vi "OE2031&OE2041_Configure Auto_Setting.vi"(7 "OE2041_Auto Setting":T1, 8 "Error in (no error)":errorcluster caption="error out（no error）", 9 "Remote Mode":u16(ring) items=["USB"=0, "RS232"=1, "Ethernet"=3], 10 "Connection ID in":refnum<k5>, 11 "VISA resource name":refnum<visa-resource-name>) -> (0 "Error out":errorcluster caption="error out", 1 "Output String":string, 2 "Connection ID out":refnum<k5>, 3 "VISA resource  out":refnum<visa-resource-name>)   [LabVIEW 2011]
panel:
  out "字符串":string
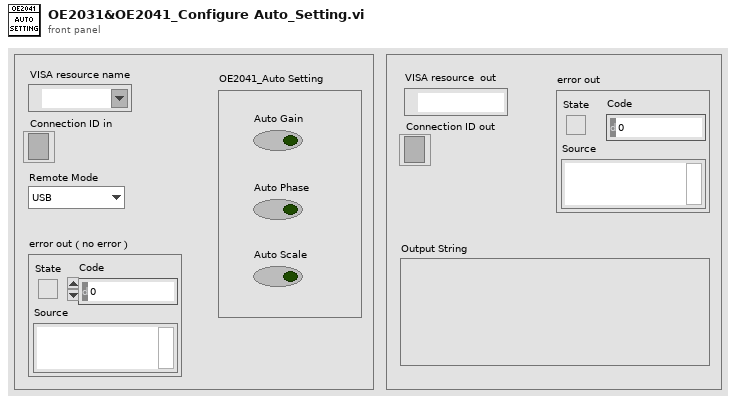
[diagram p1: front panel]
types:
  T1 = cluster{"Auto Gain":bool, "Auto Phase":bool, "Auto Scale":bool}
  T2 = enum16{"ISRC", "IGND", "ICPL", "ILIN", "PHAS", "FMOD", "RSLP", "FREQ", "SWPT", "SLLM", "SULM", "SSLL", "SSLG", "STLM", "SWRM", "IRNG", "SENS", "RMOD", "OFLT", "OFSL", "SYNC", "DMOD", "HARM", "DARB", "SWVT", "SLVL", "SVLL", "SVUL", "SVSL", "SVSG", "SVTM", "SVRM", "RALL", "SNAP", "OUTP", "OAUX", "COUT", "CAUX", "COFP", "CEXP", "FPOP", "OEXP", "*IDN", "*RST", "OVLD", "INOV", "GNOV", "*PLL", "SSET", "RSET", "AGAN", "APHS", "ARSV", "ASCL", "EQCD", "EQCS", "SPED", "SRAT", "SLEN", "SSLE", "STRG", "SPRM", "STRD", "PAUS", "REST", "SPTS", "TRCA", "TEMP", "RSTU", "IHNZ", "DEQU", "SADD", "ARNG", "CSPE", "ISRCD", "IGNDD", "ICPLD", "ILIND", "PHASD", "FMODD", "RSLPD", "FREQD", "SWPTD", "SLLMD", "SULMD", "SSLLD", "SSLGD", "STLMD", "SWRMD", "SENSD", "RMODD", "OFLTD", "OFSLD", "SYNCD", "HARMD", "EQCDD", "EQCSD", "SNAPD", "OUTPD", "SWVTD", "SLVLD", "SVLLD", "SVULD", "SVSLD", "SVSGD", "SVTMD", "SVRMD", "SVDCD", "ARSVD", "AGAND", "APHSD", "ASCLD", "FPOPD", "CAUXD", "OEXPD", "SPEDD", "SRATD", "SLEND", "SSLED", "STRGD", "SPRMD", "STRDD", "PAUSD", "RESTD", "SPTSD", "TRCAD", "*IDND", "*RSTD", "INOVD", "GNOVD", "*PLLD", "SSETD", "RSETD"}
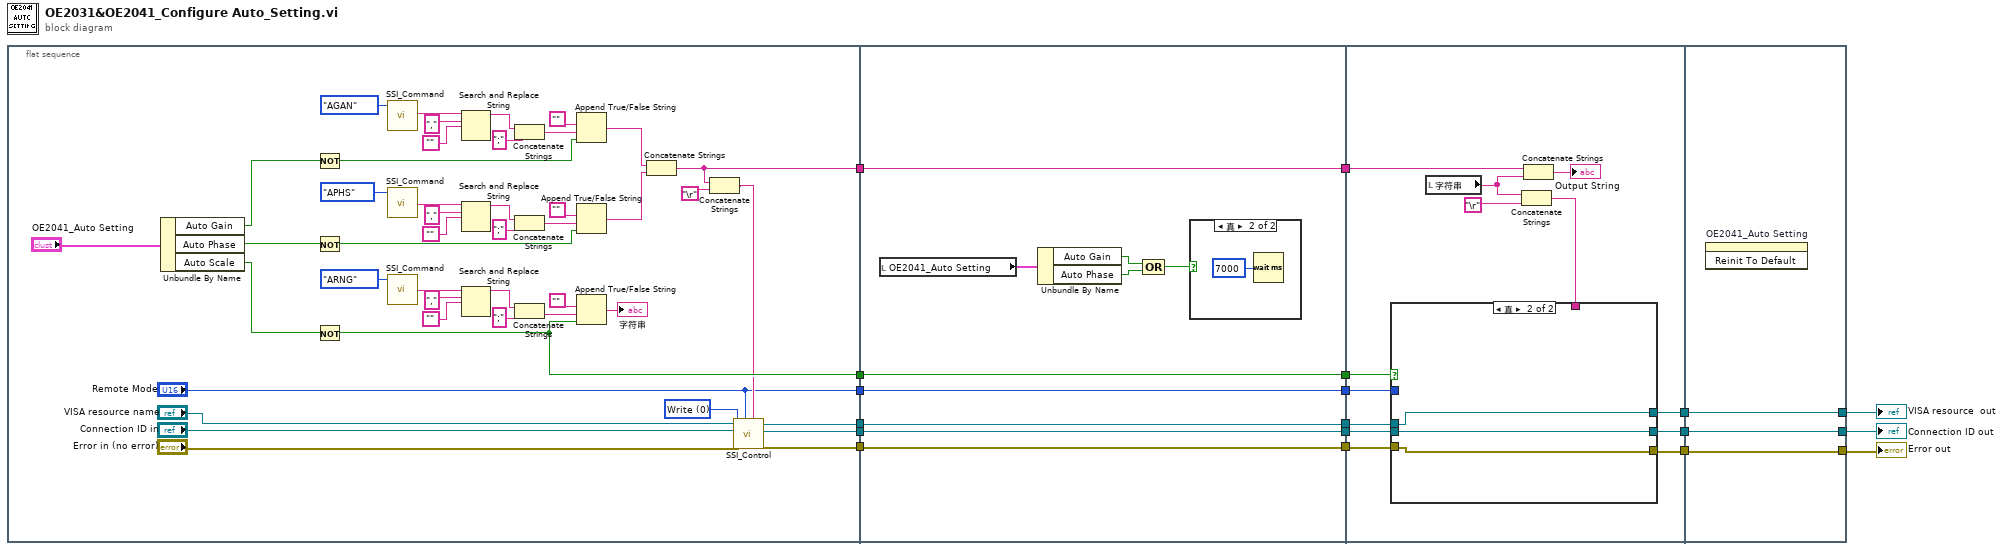
[diagram p0: block diagram]
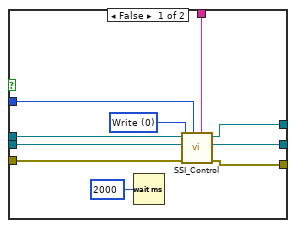
[diagram p3: hidden frame]
diagram:
  n1 = flat-sequence {
    tunnel: [w59] -> w18
    tunnel: [w58] -> w17
    tunnel: [w57] -> w16
    tunnel: [w25] -> w11
    tunnel: [w20] -> w7
    tunnel: ["Remote Mode"] -> w5
    tunnel: w18 -> [w73]
    tunnel: w17 -> [w72]
    tunnel: w16 -> [w71]
    tunnel: [w73] -> w15
    tunnel: [w72] -> w14
    tunnel: [w71] -> w13
    tunnel: [w66] -> w12
    tunnel: w11 -> [w66]
    tunnel: w7 -> [w65]
    tunnel: [w65] -> w6
    tunnel: w5 -> [w64]
    tunnel: [w64] -> w4
    tunnel: w15 -> [w85]
    tunnel: w14 -> [w86]
    tunnel: w13 -> [w84]
    tunnel: w12 -> [w87]
    tunnel: w6 -> [w79]
    tunnel: w4 -> [w78]
    tunnel: [w83] -> w3
    tunnel: [w82] -> w2
    tunnel: [w81] -> w1
    tunnel: [w101] -> w8
    tunnel: [w102] -> w9
    tunnel: [w103] -> w10
    tunnel: w3 -> [w103]
    tunnel: w2 -> [w102]
    tunnel: w1 -> [w101]
    frame #0 {
      w60 = u16 0 items=["Write", "Read"] ("Control")
      n2 = Unbundle By Name("OE2041_Auto Setting") -> ("Auto Gain"=w26:bool, "Auto Phase"=w29:bool, "Auto Scale"=w30:bool)
      n3 = Not(x=w26) -> (.not. x?=w27:bool)
      n4 = Not(x=w29) -> (.not. x?=w28:bool)
      n5 = Not(x=w30) -> (.not. x?=w25:bool)
      n6 = call "SSI_Command.vi"("Command Type"=T2."AGAN") -> ("Output string"=w33:string)  [unwired: 3 in]
      n7 = call "SSI_Command.vi"("Command Type"=T2."APHS") -> ("Output string"=w35:string)  [unwired: 3 in]
      n8 = call "SSI_Command.vi"("Command Type"=T2."ARNG") -> ("Output string"=w34:string)  [unwired: 3 in]
      n9 = Search and Replace String(input string=w33, search string="," ("搜索字符串"), replace string="") -> (result string=w45:string)  [unwired: 5 in, 3 out]
      n10 = Search and Replace String(input string=w35, search string="," ("搜索字符串"), replace string="") -> (result string=w42:string)  [unwired: 5 in, 3 out]
      n11 = Search and Replace String(input string=w34, search string="," ("搜索字符串"), replace string="") -> (result string=w39:string)  [unwired: 5 in, 3 out]
      n12 = Concatenate Strings(w45, ";") -> (w38:string)
      n13 = Concatenate Strings(w42, ";") -> (w37:string)
      n14 = Concatenate Strings(w39, ";") -> (w36:string)
      n15 = Append True/False String(1:w27, 2:w38, 3:"") -> (0:w24:string)  [unwired: 1 in]
      n16 = Append True/False String(1:w28, 2:w37, 3:"") -> (0:w23:string)  [unwired: 1 in]
      n17 = Append True/False String(1:w25, 2:w36, 3:"") -> (0:→"字符串":string)  [unwired: 1 in]
      n18 = Concatenate Strings(w24, w23) -> (w20:string)
      n19 = Concatenate Strings(w20, "\r") -> (w21:string)
      n20 = call "SSI_Control.vi"("Write Buffer"=w21, "Remote Mode"="Remote Mode", "Error in (no error)"="Error in (no error)", "Control"=w60, "Connection ID in"="Connection ID in", "VISA resource name"="VISA resource name") -> ("Error out"=w57:errorcluster, "Connection ID out"=w59:refnum<k5>, "VISA resource  out"=w58:refnum<visa-resource-name>)  [unwired: 2 in, 1 out]
    }
    frame #1 {
      n21 = local read "OE2041_Auto Setting"() -> (w67:T1)
      n22 = Unbundle By Name(w67) -> ("Auto Gain"=w69:bool, "Auto Phase"=w68:bool)
      n23 = Compound Arithmetic op=OR(w69, w68) -> (w70:bool)
      n24 = case shown="真" w70 {
        frame False {
        }
        frame True {
          n25 = Wait (ms)(milliseconds to wait=u32 7000 ("等待时间（毫秒）")) -> ()  [unwired: 1 out]
        }
      }
    }
    frame #2 {
      n26 = local read "字符串"() -> (w77:string)
      n27 = Concatenate Strings(w77, "\r") -> (w75:string)
      n28 = case shown="真" w87 {
        tunnel: w86 -> [w96 w100]
        tunnel: w85 -> [w95 w99]
        tunnel: w84 -> [w94 w98]
        tunnel: [w93 w98] -> w83
        tunnel: [w92 w99] -> w82
        tunnel: [w91 w100] -> w81
        tunnel: w75 -> [w89 _]
        tunnel: w78 -> [w88 _]
        frame False {
          w97 = u16 0 items=["Write", "Read"] ("Control")
          n29 = Wait (ms)(milliseconds to wait=u32 2000 ("等待时间（毫秒）")) -> ()  [unwired: 1 out]
          n30 = call "SSI_Control.vi"("Write Buffer"=w89, "Remote Mode"=w88, "Error in (no error)"=w94, "Control"=w97, "Connection ID in"=w95, "VISA resource name"=w96) -> ("Error out"=w93:errorcluster, "Connection ID out"=w92:refnum<k5>, "VISA resource  out"=w91:refnum<visa-resource-name>)  [unwired: 2 in, 1 out]
        }
        frame True {
        }
      }
      n31 = Concatenate Strings(w79, w77) -> (→"Output String":string)
    }
    frame #3 {
      n32 = invoke on="OE2041_Auto Setting" class="Clust (严格)" method="Reinit To Default"() -> ()  [unwired: 3 in, 3 out]
    }
  }
  "Error out" <- w10
  "Connection ID out" <- w9
  "VISA resource  out" <- w8
